vi "GPR Configuration.vi"(8 "error in (no error)":errorcluster, 11 "GPR Graph Info In":T1={"Display Type"=enum."Wiggle Trace", "Display Info"={"X Scale"={"X Scale Label"=FALSE, "X Scale Name"="", "X Scale Visible"=FALSE, "dx"=0.0}, "Y Scale"={"X Scale Label"=FALSE, "X Scale Name"="", "X Scale Visible"=FALSE, "dt"=0.0}, "BackGround Color"=0}, "Trace Options"={"Trace Amplitude"=0.0, "Trace Color"=0, "Fill options"=enum."No Fill"}, "Intensity Options"={"Color Scale"=enum."RGB"}}) -> (0 "error out":errorcluster, 3 "GPR Graph Info Out":T1={"Display Type"=enum."Wiggle Trace", "Display Info"={"X Scale"={"X Scale Label"=FALSE, "X Scale Name"="", "X Scale Visible"=FALSE, "dx"=0.0}, "Y Scale"={"X Scale Label"=FALSE, "X Scale Name"="", "X Scale Visible"=FALSE, "dt"=0.0}, "BackGround Color"=0}, "Trace Options"={"Trace Amplitude"=0.0, "Trace Color"=0, "Fill options"=enum."No Fill"}, "Intensity Options"={"Color Scale"=enum."RGB"}})   [LabVIEW 2009]
doc: "Displays a configuration dialog to configure the graph options of a GPR graph."
uses:
  Controls/Display Types.ctl
  Controls/Fill Options.ctl
  Controls/GPR Graph Info.ctl
  Controls/Display Info.ctl
  Controls/Trace Options.ctl
  Controls/Intensity Options.ctl
  Controls/Color Scales.ctl
panel:
  in  "Cancel":bool
  in  "OK":bool
  in  "Tab Control":T8(tab)=enum."Trace Plot"
  in  "Display Type":T2
  in  "Fill Options":T5
  in  "Trace Color":u32(colorbox)
  in  "BackGround Color":u32(colorbox)=16777215
  in  "Trace Amplitude":dbl=1.0
  in  "Color Scale":u16(ring)=1 items=["Blue<Green<Red", "Blue<White<Red", "Red<Green<Blue", "Red<White<Blue", "White<Grey<Black", "Black<Grey<White"]
  in  "dx":dbl=4e-10
  in  "Y Scale Visible":bool
  in  "Y Scale Name":string
  in  "Y Scale Label":bool
  in  "dt":dbl=4e-10
  in  "X Scale Visible":bool
  in  "X Scale Name":string
  in  "X Scale Label":bool
  # "Multiples of dx"
  # "Y Scale"
  # "X Scale"
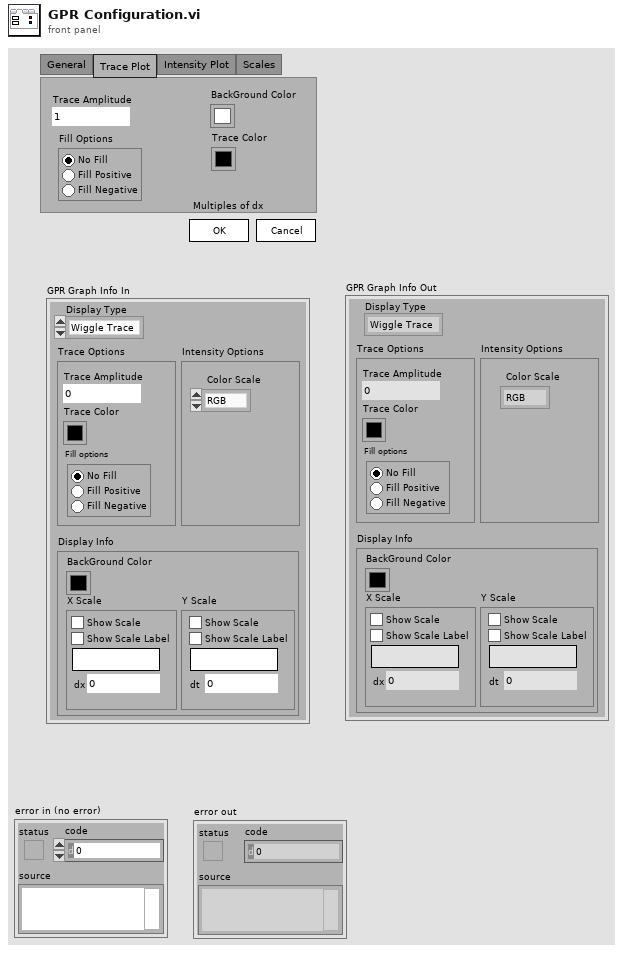
[diagram p1: front panel]
types:
  T1 = typedef "GPR Graph Info.ctl" = cluster{"Display Type":T2, "Display Info":T3, "Trace Options":T4, "Intensity Options":T6}
  T2 = typedef "Display Types.ctl" = enum16{"Intensity Plot", "Wiggle Trace"}
  T3 = typedef "Display Info.ctl" = cluster{"X Scale":cluster{"X Scale Label":bool, "X Scale Name":string, "X Scale Visible":bool, "dx":dbl}, "Y Scale":cluster{"X Scale Label":bool, "X Scale Name":string, "X Scale Visible":bool, "dt":dbl}, "BackGround Color":u32}
  T4 = typedef "Trace Options.ctl" = cluster{"Trace Amplitude":dbl, "Trace Color":u32, "Fill options":T5}
  T5 = typedef "Fill Options.ctl" = enum32{"No Fill", "Fill Positive", "Fill Negative"}
  T6 = typedef "Intensity Options.ctl" = cluster{"Color Scale":T7}
  T7 = typedef "Color Scales.ctl" = enum16{"RGB", "RWB", "BGR", "BWR", "BW", "WB"}
  T8 = enum32{"General", "Trace Plot", "Intensity Plot", "Scales"}
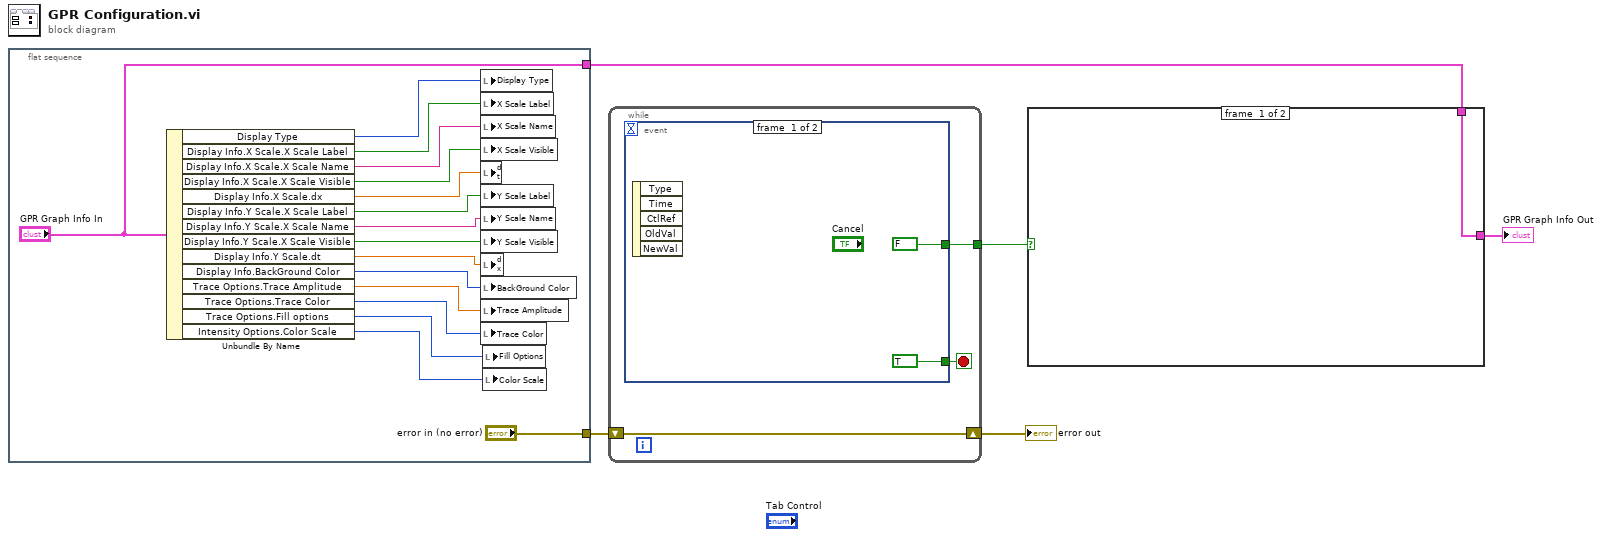
[diagram p0: block diagram]
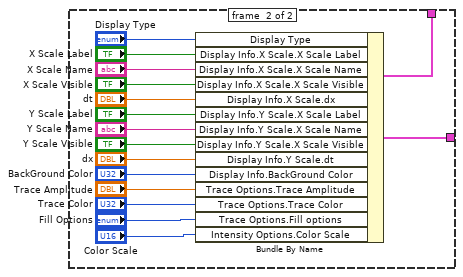
[diagram p2: hidden frame]
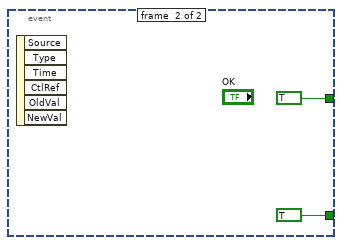
[diagram p3: hidden frame]
diagram:
  n1 = flat-sequence {
    tunnel: ["GPR Graph Info In"] -> w5
    tunnel: ["error in (no error)"] -> w3
    frame #0 {
      n2 = Unbundle By Name("GPR Graph Info In") -> ("Display Type"=w20:T2, "Display Info.X Scale.X Scale Label"=w18:bool, "Display Info.X Scale.X Scale Name"=w17:string, "Display Info.X Scale.X Scale Visible"=w16:bool, "Display Info.X Scale.dx"=w15:dbl, "Display Info.Y Scale.X Scale Label"=w21:bool, "Display Info.Y Scale.X Scale Name"=w11:string, "Display Info.Y Scale.X Scale Visible"=w12:bool, "Display Info.Y Scale.dt"=w13:dbl, "Display Info.BackGround Color"=w14:u32, "Trace Options.Trace Amplitude"=w19:dbl, "Trace Options.Trace Color"=w7:u32, "Trace Options.Fill options"=w8:T5, "Intensity Options.Color Scale"=w9:T7)
      n3 = local write "Display Type"(w20) -> ()
      n4 = local write "X Scale Label"(w18) -> ()
      n5 = local write "X Scale Name"(w17) -> ()
      n6 = local write "X Scale Visible"(w16) -> ()
      n7 = local write "dt"(w15) -> ()
      n8 = local write "Y Scale Label"(w21) -> ()
      n9 = local write "Y Scale Name"(w11) -> ()
      n10 = local write "Y Scale Visible"(w12) -> ()
      n11 = local write "dx"(w13) -> ()
      n12 = local write "BackGround Color"(w14) -> ()
      n13 = local write "Trace Amplitude"(w19) -> ()
      n14 = local write "Trace Color"(w7) -> ()
      n15 = local write "Fill Options"(w8) -> ()
      n16 = local write "Color Scale"(w9) -> ()
    }
  }
  n17 = while {
    tunnel: [w24] -> w4
    shift-right: [w22] -> w2
    shift-left: w3 -> [w22]
    stop <- w23 stop-if-true
    n18 = event shown="[1] \"OK\": Value Change" {
      selector: _ -> [_ _]
      dyn-events: _ -> [_ _]
      timeout: _ -> [_ _]
      tunnel: [FALSE ("Cancel") TRUE ("Cancel")] -> w24
      tunnel: [TRUE TRUE] -> w23
      event #0 {
        n19 = event-data() -> ()  [unwired: 1 in, 5 out]
      }
      event #1 {
        n20 = event-data() -> ()  [unwired: 1 in, 6 out]
      }
    }
  }
  "error out" <- w2
  n21 = case shown="True" w4 {
    tunnel: [w29 w45] -> w1
    tunnel: w5 -> [w29 w44]
    frame #0 {
    }
    frame #1 {
      n22 = Bundle By Name(cluster=w44, "Display Type"="Display Type", "Display Info.X Scale.X Scale Label"="X Scale Label", "Display Info.X Scale.X Scale Name"="X Scale Name", "Display Info.X Scale.X Scale Visible"="X Scale Visible", "Display Info.X Scale.dx"="dt", "Display Info.Y Scale.X Scale Label"="Y Scale Label", "Display Info.Y Scale.X Scale Name"="Y Scale Name", "Display Info.Y Scale.X Scale Visible"="Y Scale Visible", "Display Info.Y Scale.dt"="dx", "Display Info.BackGround Color"="BackGround Color", "Trace Options.Trace Amplitude"="Trace Amplitude", "Trace Options.Trace Color"="Trace Color", "Trace Options.Fill options"="Fill Options", "Intensity Options.Color Scale"="Color Scale") -> (w45:T1)
    }
  }
  "GPR Graph Info Out" <- w1
